vi "MsgMyMessage.vi"() -> (1 "MessageName":string)   [LabVIEW 2017, in "Loop7.lvlib"]
uses:
  <vilib>/addons/InsightCM/Devices/Shared/Common/DataFlow/test/SpeedBenchmark/Loop7/Loop7.lvlib
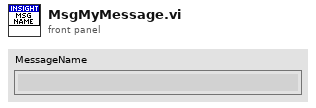
[diagram p1: front panel]
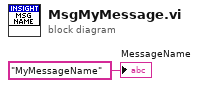
[diagram p0: block diagram]
diagram:
  "MessageName" <- "MyMessageName" ("ProcessName")
